vi "Configure List SAV Or RCL.vi"(8 "error in (no error)":errorcluster, 9 "Save Type ( 0 : Save)":u16(ring) caption="Save Type" items=["Save", "RCL"], 10 "File Add ( 1 - 5 )":u32=1, 11 "VISA resource name":refnum<visa-resource-name>) -> (0 "error out":errorcluster, 3 "VISA resource name out":refnum<visa-resource-name>)   [LabVIEW 2015, in "IT8900A-E.lvlib"]
doc: "This command stores the list file of the current load to the specified location of the storage.Up to 5 files can be stored, and the files saved in 1-5 are not easy to lose. When the power is off, the data is saved.\n\n<b>Save Type</b>\n0:Save : The order restores a LIST file that is currently stored in memory to a specified location with a LIST:SAV command.\n1:RCL : This command invokes an existing sequential file directly with a LIST:RCL command."
uses:
  <instrlib>/IT8900/IT8900A-E.lvlib
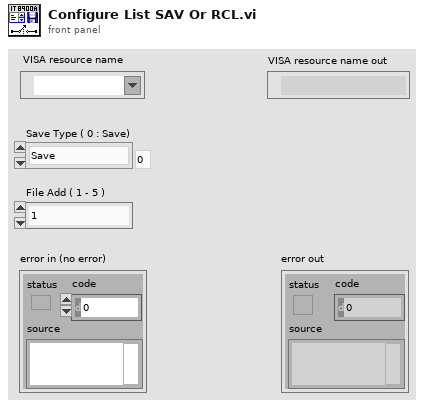
[diagram p1: front panel]
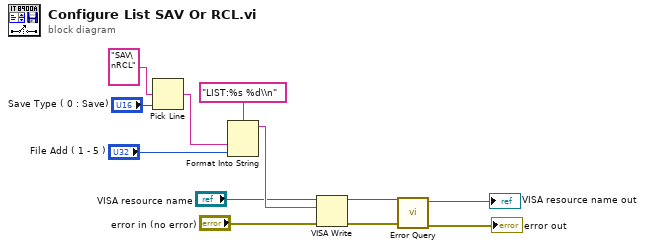
[diagram p0: block diagram]
diagram:
  n1 = Pick Line(multi-line string="SAV\nRCL", line index="Save Type ( 0 : Save)") -> (output string=w1:string)  [unwired: 1 in]
  n2 = Format Into String(format string="LIST:%s %d\\n", w1, "File Add ( 1 - 5 )") -> (resulting string=w11:string)  [unwired: 2 in, 1 out]
  n3 = VISA Write(VISA resource name="VISA resource name", write buffer=w11, error in (no error)="error in (no error)") -> (VISA resource name out=w8:refnum<visa-resource-name>, error out=w6:errorcluster)  [unwired: 1 out]
  n4 = call <instrlib>:"Error Query.vi"("error in (no error)"=w6, "VISA resource name"=w8) -> ("error out"=→"error out":errorcluster, "VISA resource name out"=→"VISA resource name out":refnum<visa-resource-name>)  [unwired: 6 in, 2 out]
